vi "_Parse Detected Allocation.vi"(8 "error in (no error)":errorcluster, 10 "Input String":string, 11 "VISA resource name":refnum<visa-resource-name>) -> (0 "error out":errorcluster, 1 "Detected Allocation":T1, 2 "Reliability":i32, 3 "VISA resource name out":refnum<visa-resource-name>)   [LabVIEW 2020, in "Rohde&Schwarz CMWXP NR FR1 Measurement.lvlib"]
uses:
  <instrlib>/Rohde&Schwarz CMWXP NR FR1 Measurement/Rohde&Schwarz CMWXP NR FR1 Measurement.lvlib
  <instrlib>/Rohde&Schwarz CMWXP NR FR1 Measurement/Private/rsidr_core.llb/rsidr_core.lvlib
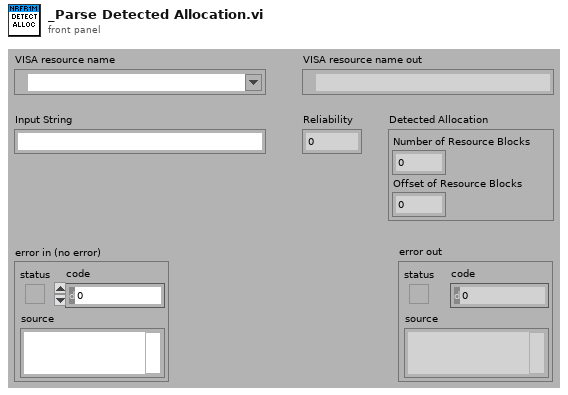
[diagram p1: front panel]
types:
  T1 = cluster{"Number of Resource Blocks":i32, "Offset of Resource Blocks":i32}
  T2 = cluster{"Nr Res Blocks":i32, "Offset Res Blocks":i32}
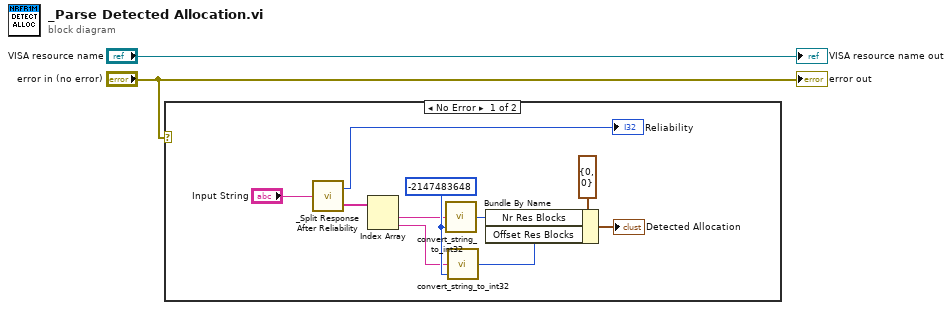
[diagram p0: block diagram]
diagram:
  n1 = case shown="No Error" "error in (no error)" {
    frame No Error {
      w12 = -2147483648
      n2 = call <instrlib>:"_Split Response After Reliability.vi"("Input String"="Input String") -> ("Response out"=w7:string[], "Reliability out"=→"Reliability":i32)
      n3 = Index Array(array=w7) -> (element #1=w4:string, element #2=w3:string)  [unwired: 2 in]
      n4 = call <instrlib>:"convert_string_to_int32.vi"("default (0)"=w12, "String in"=w4) -> ("int32 value out"=w9:i32)  [unwired: 3 in]
      n5 = call <instrlib>:"convert_string_to_int32.vi"("default (0)"=w12, "String in"=w3) -> ("int32 value out"=w8:i32)  [unwired: 3 in]
      n6 = Bundle By Name(cluster=T2 {"Nr Res Blocks"=0, "Offset Res Blocks"=0} ("Detected Allocation"), "Nr Res Blocks"=w9, "Offset Res Blocks"=w8) -> (→"Detected Allocation":T2)
    }
    frame Error {
    }
  }
  "VISA resource name out" <- "VISA resource name"
  "error out" <- "error in (no error)"
